vi "TEST From To String.vi"() -> ()   [LabVIEW 2013, in "Carya Config.lvclass"]
doc: "Copyright 2018, Carya Automatisering, Wiebe Walstra."
uses:
  Carya Config.lvclass
  CConfig Object/Data.ctl
  CConfig Object/CConfig Object.lvclass
panel:
  out "Context":string[](array[string])
  out "Section names":string[](array[string])
  out "Created session?":bool
  out "Created key?":bool
  out "String 3":string
  out "String 2":string
  out "Equal?":bool
  out "String":string
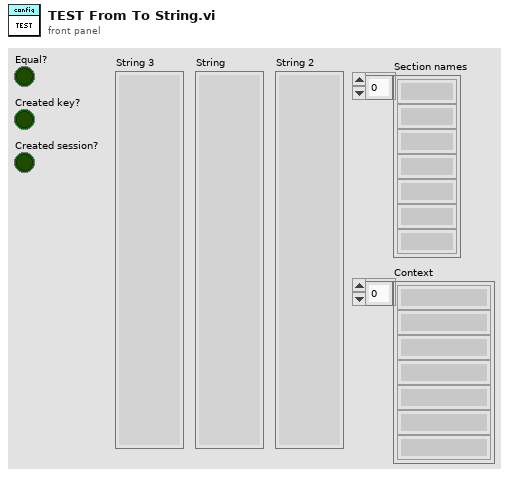
[diagram p1: front panel]
types:
  T1 = typedef "CConfig Object.lvclass/Data.ctl" = enum16{"pre", "name", "middle", "value", "post", "newline", "persistant", "tagged", "type"}
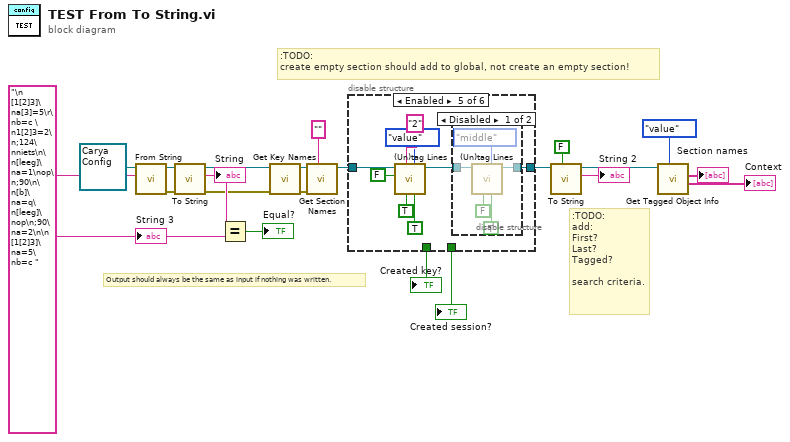
[diagram p0: block diagram]
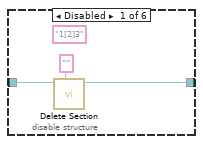
[diagram p2: hidden frame]
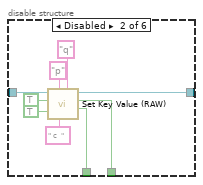
[diagram p3: hidden frame]
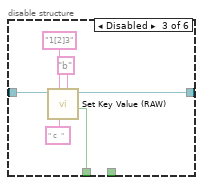
[diagram p4: hidden frame]
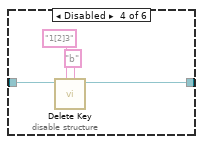
[diagram p5: hidden frame]
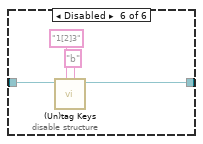
[diagram p7: hidden frame]
diagram:
  w10 = "\n [1[2]3]\na[3]=5\r\nb=c \n1[2]3=2\n;124\nniets\n\n[leeg]\na=1\nop\n;90\n\n[b]\na=q\n[leeg]\nop\n;90\na=2\n\n [1[2]3]\na=5\nb=c " ("String")
  # ":TODO:\nadd:\nFirst?\nLast?\nTagged?\n\nsearch criteria."
  # ":TODO:\ncreate empty section should add to global, not create an empty section!"
  # "Output should always be the same as input if nothing was written."
  n1 = call-dynamic "From String.vi"("String"=w10, "Carya Config in"=refnum<class "Carya Config.lvclass"> refnum) -> ("error out"=w16:errorcluster, "Carya Config out"=w21:refnum<class "Carya Config.lvclass">)  [unwired: 7 in, 1 out]
  n2 = call-dynamic "To String.vi"("error in (no error)"=w16, "Carya Config in"=w21) -> ("error out"=w15:errorcluster, "String"=w20:string, "Carya Config out"=w18:refnum<class "Carya Config.lvclass">)  [unwired: 7 in]
  "String" <- w20
  n3 = Equal?(x=w20, y=w10) -> (x = y?=→"Equal?":bool)
  n4 = call-dynamic "Get Key Names.vi"("error in (no error)"=w15, "Carya Config in"=w18) -> ("error out"=w14:errorcluster, "Carya Config out"=w17:refnum<class "Carya Config.lvclass">)  [unwired: 5 in, 3 out]
  n5 = call-dynamic "Get Section Names.vi"("Section Regex [\"\", all]"="" ("Section Regex [\"\", all]"), "error in (no error)"=w14, "Carya Config in"=w17) -> ("Carya Config out"=w11:refnum<class "Carya Config.lvclass">)  [unwired: 6 in, 2 out]
  n6 = disable-structure shown="Enabled" {
    disable-tunnel: [w24 w32 w38 w42 w45 w60] -> w13
    disable-tunnel: w11 -> [w22 w33 w39 w43 w51 w61]
    disable-tunnel: [_ w28 w34 _ _ _] -> w7
    disable-tunnel: [_ w25 _ _ _ _] -> w6
    frame Disabled {
      (unwired) "1[2]3" ("Section name")
      n7 = call-dynamic "Delete Section.vi"("Section name"="", "Carya Config in"=w22) -> ("Carya Config out"=w24:refnum<class "Carya Config.lvclass">)  [unwired: 7 in, 2 out]
    }
    frame Disabled {
      n8 = call-dynamic "Set Key Value (RAW).vi"("Key name"="q", "Key value"=" c  ", "Section name"="p", "Create key? [T]"=TRUE, "Create section? [T]"=TRUE, "Carya Config in"=w33) -> ("Created key?"=w28:bool, "Created session?"=w25:bool, "Carya Config out"=w32:refnum<class "Carya Config.lvclass">)  [unwired: 1 in, 2 out]
    }
    frame Disabled {
      n9 = call-dynamic "Set Key Value (RAW).vi"("Key name"="b", "Key value"=" c  ", "Section name"="1[2]3", "Carya Config in"=w39) -> ("Created key?"=w34:bool, "Carya Config out"=w38:refnum<class "Carya Config.lvclass">)  [unwired: 3 in, 3 out]
    }
    frame Disabled {
      n10 = call-dynamic "Delete Key.vi"("Key name"="b", "Section name"="1[2]3", "Carya Config in"=w43) -> ("Carya Config out"=w42:refnum<class "Carya Config.lvclass">)  [unwired: 5 in, 3 out]
    }
    frame Enabled {
      n11 = call-dynamic "(Un)tag Lines.vi"("Set if match (T)\\Set it no match (F) [T]"=TRUE ("Set if match (T)\\Set it no match (F) [T]"), "Context [name]"=Data."value", "Tag (T)\\Untag (F) [T]"=TRUE ("Tag (T)\\Untag (F) [T]"), "String\\Regex [\"\"]"="2" ("Section name"), "Use Regex? [T]"=FALSE, "Carya Config in"=w51) -> ("Carya Config out"=w46:refnum<class "Carya Config.lvclass">)  [unwired: 2 in, 3 out]
      n12 = disable-structure shown="Disabled" {
        disable-tunnel: w46 -> [w56 w57]
        disable-tunnel: [w55 w57] -> w45
        frame Disabled {
          n13 = call-dynamic "(Un)tag Lines.vi"("Set if match (T)\\Set it no match (F) [T]"=TRUE ("Set if match (T)\\Set it no match (F) [T]"), "Context [name]"=Data."middle", "Tag (T)\\Untag (F) [T]"=FALSE ("Tag (T)\\Untag (F) [T]"), "Carya Config in"=w56) -> ("Carya Config out"=w55:refnum<class "Carya Config.lvclass">)  [unwired: 4 in, 3 out]
        }
        frame Enabled {
        }
      }
    }
    frame Disabled {
      n14 = call-dynamic "(Un)tag Keys.vi"("Key name/Regex"="b" ("Key name"), "Section name/Regex"="1[2]3" ("Section name"), "Carya Config in"=w61) -> ("Carya Config out"=w60:refnum<class "Carya Config.lvclass">)  [unwired: 7 in, 1 out]
    }
  }
  "Created key?" <- w7
  "Created session?" <- w6
  n15 = call-dynamic "To String.vi"("Persitant only? [T]"=FALSE ("Persitant only?"), "Carya Config in"=w13) -> ("String"=→"String 2":string, "Carya Config out"=w5:refnum<class "Carya Config.lvclass">)  [unwired: 7 in, 1 out]
  n16 = call-dynamic "Get Tagged Object Info.vi"("Context [name]"=Data."value", "Carya Config in"=w5) -> ("Context"=→"Context":string[], "Section names"=→"Section names":string[])  [unwired: 6 in, 2 out]
  "String 3" <- w10
